vi "WriteCurrentTime.vi"(8 "error in (no error)":errorcluster, 9 "TimeString":string, 10 "Start\\End":string, 11 "refnum out":refnum<file>) -> (0 "error out":errorcluster, 3 "refnum out 2":refnum<file>)   [LabVIEW 2012]
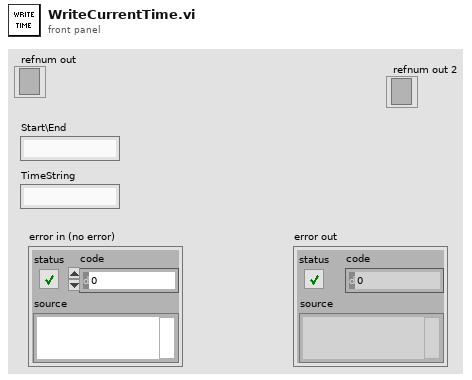
[diagram p1: front panel]
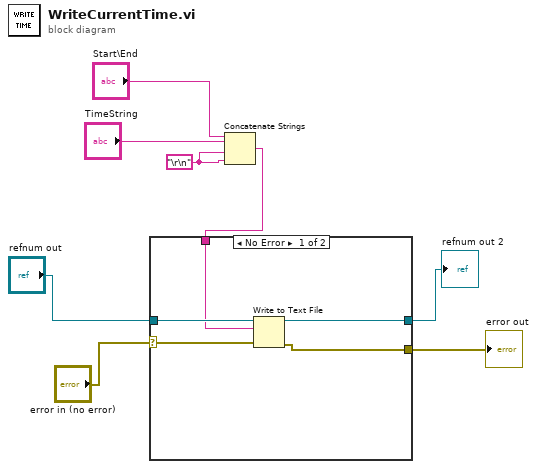
[diagram p0: block diagram]
diagram:
  w1 = "\r\n"
  n1 = Concatenate Strings("Start\\End", "TimeString", w1, w1) -> (w4:string)
  n2 = case shown="No Error" "error in (no error)" {
    selector: "error in (no error)" -> [w12 w14]
    tunnel: [w11 w14] -> w7
    tunnel: "refnum out" -> [w13 _]
    tunnel: w4 -> [w10 _]
    tunnel: [w9 _] -> w5
    frame No Error {
      n3 = Write to Text File(file (use dialog)=w13, text=w10, error in=w12) -> (refnum out=w9:refnum<file>, error out=w11:errorcluster)  [unwired: 1 in, 1 out]
    }
    frame Error {
    }
  }
  "error out" <- w7
  "refnum out 2" <- w5
